vi "while loop 10.vi"() -> ()   [LabVIEW 2025]
panel:
  in  "stop":bool
  in  "Numeric":dbl
  in  "Slide":dbl(slide) scale=0.0..10.0
  out "Tank":dbl(slide) scale=0.0..20.0
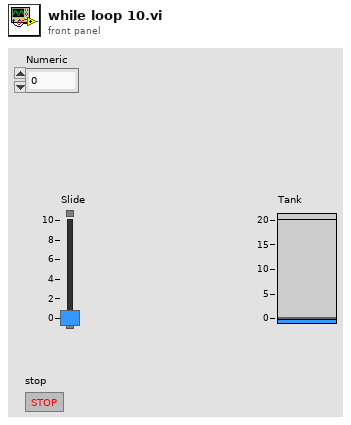
[diagram p1: front panel]
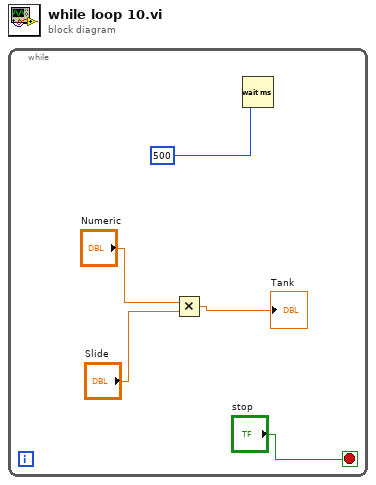
[diagram p0: block diagram]
diagram:
  n1 = while {
    stop <- "stop" stop-if-true
    n2 = Multiply(x="Numeric", y="Slide") -> (x*y=→"Tank":dbl)
    n3 = Wait (ms)(milliseconds to wait=500) -> ()  [unwired: 1 out]
  }
